vi "Build Event Log Path.vi"(8 "error in (no error)":errorcluster, 11 "Text File Sink in":refnum<class "Text File Sink.lvclass">) -> (0 "error out":errorcluster, 3 "Text File Sink out":refnum<class "Text File Sink.lvclass">)   [LabVIEW 2016, in "Stream Log.lvlib" / "Text File Sink.lvclass"]
doc: "--\nCopyright © 2017 Composed SystemsI All rights reserved.\n\nAuthor: Jon McBee <jon.mcbee@composed.io>\n\nThis library is provided \"AS IS\" ,WITHOUT WARRANTIES OR\nCONDITIONS OF ANY KIND, either express or implied.\n\nComposed Systems -- composed.io\n\nStream 0.0.1.1\nJon McBee - Composed Systems\nCopyright (c) 2017, Composed Systems"
uses:
  <userlib>/Composed Systems/Stream/Log/Text File Sink/Text File Sink.lvclass
  <userlib>/Composed Systems/Stream/Log/Text File Sink/Text File Sink.lvclass/Text File Sink.ctl
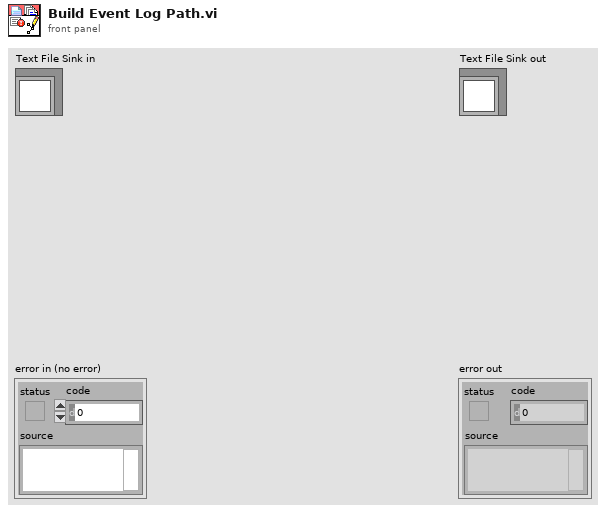
[diagram p1: front panel]
types:
  T1 = typedef "LVDateTimeRec.ctl" = cluster{"fractional second":dbl, "second":i32, "minute":i32, "hour":i32, "day of month":i32, "month":i32, "year":i32, "day of week":i32, "day of year":i32, "DST":i32}
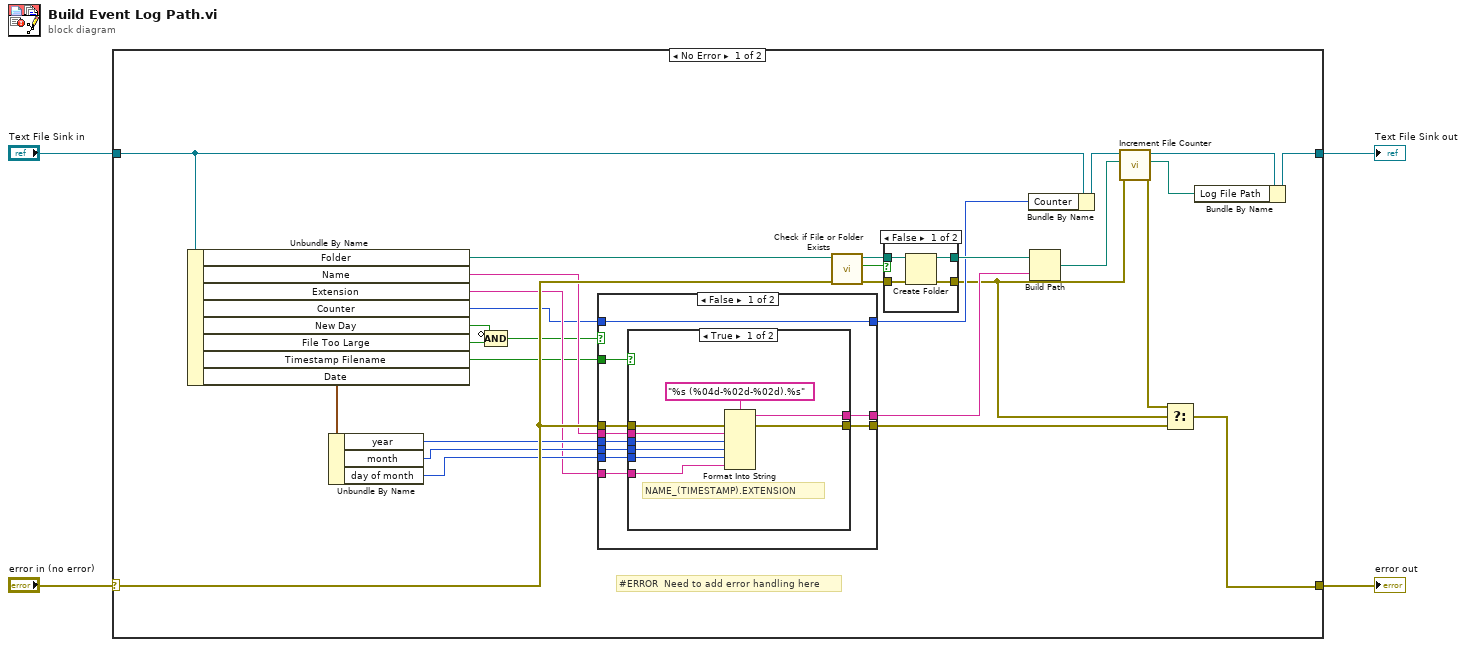
[diagram p0: block diagram]
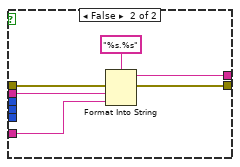
[diagram p2: hidden frame]
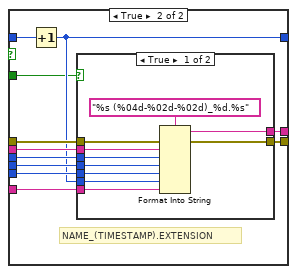
[diagram p3: hidden frame]
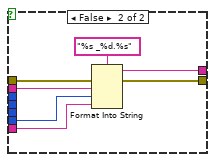
[diagram p4: hidden frame]
diagram:
  n1 = case shown="No Error" "error in (no error)" {
    selector: "error in (no error)" -> [w26 w94]
    tunnel: [w14 w94] -> w3
    tunnel: [w15 w93] -> w1
    tunnel: "Text File Sink in" -> [w13 w93]
    frame No Error {
      # "#ERROR  Need to add error handling here"
      n2 = Unbundle By Name(w13) -> ("Folder"=w27:path, "Name"=w24:string, "Extension"=w20:string, "Counter"=w19:u16, "New Day"=w17:bool, "File Too Large"=w18:bool, "Timestamp Filename"=w5:bool, "Date"=w25:T1)
      n3 = Unbundle By Name(w25) -> ("year"=w23:i32, "month"=w22:i32, "day of month"=w21:i32)
      n4 = Compound Arithmetic op=AND(invert w17, w18) -> (w16:bool)
      n5 = case shown="False" w16 {
        tunnel: [w43 w69] -> w29
        tunnel: [w42 w68] -> w28
        tunnel: w26 -> [w41 w67]
        tunnel: w24 -> [w40 w66]
        tunnel: w23 -> [w39 w65]
        tunnel: w22 -> [w38 w64]
        tunnel: w21 -> [w37 w63]
        tunnel: w20 -> [w36 w62]
        tunnel: w19 -> [w35 w61]
        tunnel: [w35 w60] -> w12
        tunnel: w5 -> [w34 w59]
        frame False {
          n6 = case shown="True" w34 {
            tunnel: [w51 w57] -> w43
            tunnel: [w50 w56] -> w42
            tunnel: w41 -> [w49 w55]
            tunnel: w40 -> [w48 w54]
            tunnel: w39 -> [w47 _]
            tunnel: w38 -> [w46 _]
            tunnel: w37 -> [w45 _]
            tunnel: w36 -> [w44 w53]
            frame True {
              # "NAME_(TIMESTAMP).EXTENSION"
              n7 = Format Into String(format string="%s (%04d-%02d-%02d).%s", error in=w49, w48, w47, w46, w45, w44) -> (resulting string=w51:string, error out=w50:errorcluster)  [unwired: 1 in]
            }
            frame False {
              n8 = Format Into String(format string="%s.%s", error in=w55, w54, w53) -> (resulting string=w57:string, error out=w56:errorcluster)  [unwired: 1 in]
            }
          }
        }
        frame True {
          # "NAME_(TIMESTAMP).EXTENSION"
          n9 = Increment(x=w61) -> (x+1=w60:u16)
          n10 = case shown="True" w59 {
            tunnel: [w78 w85] -> w69
            tunnel: [w77 w84] -> w68
            tunnel: w67 -> [w76 w83]
            tunnel: w66 -> [w75 w82]
            tunnel: w65 -> [w74 _]
            tunnel: w64 -> [w73 _]
            tunnel: w63 -> [w72 _]
            tunnel: w62 -> [w71 w80]
            tunnel: w60 -> [w70 w81]
            frame True {
              n11 = Format Into String(format string="%s (%04d-%02d-%02d)_%d.%s", error in=w76, w75, w74, w73, w72, w70, w71) -> (resulting string=w78:string, error out=w77:errorcluster)  [unwired: 1 in]
            }
            frame False {
              n12 = Format Into String(format string="%s _%d.%s", error in=w83, w82, w81, w80) -> (resulting string=w85:string, error out=w84:errorcluster)  [unwired: 1 in]
            }
          }
        }
      }
      n13 = call <vilib>:"Check if File or Folder Exists.vi"("error in (no error)"=w26, "path"=w27) -> ("error out"=w31:errorcluster, "file or folder exists?"=w33:bool, "dup path"=w32:path)  [unwired: 7 out]
      n14 = case shown="False" w33 {
        tunnel: w32 -> [w89 w92]
        tunnel: w31 -> [w90 w91]
        tunnel: [w88 w91] -> w7
        tunnel: [w87 w92] -> w30
        frame False {
          n15 = Create Folder(path (use dialog)=w89, error in=w90) -> (created path=w87:path, error out=w88:errorcluster)  [unwired: 2 out]
        }
        frame True {
        }
      }
      n16 = Bundle By Name(cluster=w13, "Counter"=w12) -> (w11:refnum<class "Text File Sink.lvclass">)
      n17 = Build Path(base path=w30, name or relative path=w29) -> (appended path=w9:path)
      n18 = call <userlib>:"Increment File Counter.vi"("error in (no error)"=w7, "File Path"=w9, "Text File Sink in"=w11) -> ("error out"=w6:errorcluster, "File Path out"=w8:path, "Text File Sink out"=w10:refnum<class "Text File Sink.lvclass">)  [unwired: 6 in]
      n19 = Select(t=w6, s=w7, f=w28) -> (s? t:f=w14:errorcluster)
      n20 = Bundle By Name(cluster=w10, "Log File Path"=w8) -> (w15:refnum<class "Text File Sink.lvclass">)
    }
    frame Error {
    }
  }
  "error out" <- w3
  "Text File Sink out" <- w1
